vi "Easy Color Columns.vi"(4 "font Size(10)":sgl=10.0, 6 "BGK Color":u32(colorbox)=16766018, 8 "error in (no error)":errorcluster, 11 "DataGridView in":refnum<class "DataGridView.lvclass">) -> (0 "error out":errorcluster, 3 "DataGridView out":refnum<class "DataGridView.lvclass">)   [LabVIEW 2020, in "DataGrid.lvlib"]
doc: "Sets the background color and font size for the column headers."
uses:
  DataGrid.lvlib
  DataGridView/DataGridView.lvclass
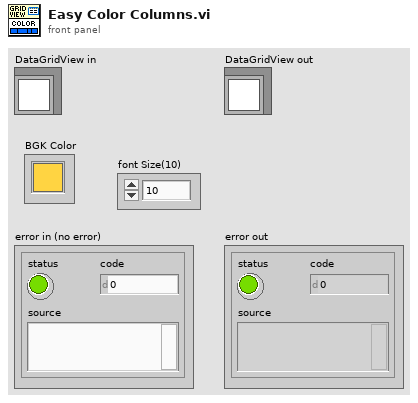
[diagram p1: front panel]
types:
  T1 = enum16{"Regular", "Bold", "Italic", "Underline", "Strikeout"}
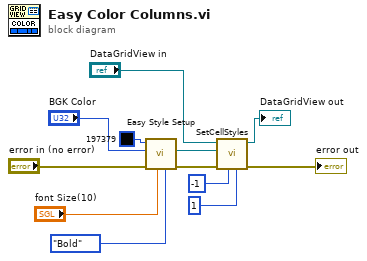
[diagram p0: block diagram]
diagram:
  n1 = call "Easy Style Setup.vi"("font style (regular)"=T1."Bold", "font Size(9)"="font Size(10)", "error in (no error)"="error in (no error)", "Color BG"="BGK Color", "Color FG"=u32 197379) -> ("error out"=w2:errorcluster, "CellStyle out"=w3:refnum<class "CellStyle.lvclass">)  [unwired: 5 in]
  n2 = call "SetCellStyles.vi"("Column"=1, "Row"=-1, "error in (no error)"=w2, "CellStyle.lvclass"=w3, "DataGridView in"="DataGridView in") -> ("error out"=→"error out":errorcluster, "DataGridView out"=→"DataGridView out":refnum<class "DataGridView.lvclass">)  [unwired: 5 in]
